vi "Build DashBoard Data.vi"(11 "Dashboard Enables":T2={"Analog Module 1"=[TRUE, TRUE, TRUE, TRUE, TRUE, TRUE, TRUE, TRUE], "Analog Module 2"=[FALSE, FALSE, FALSE, FALSE, FALSE, FALSE, FALSE, FALSE], "Digital Module 1"=TRUE, "Digital Module 2"=FALSE, "Solenoid Module"=TRUE}) -> ()   [LabVIEW 2011]
doc: "This VI builds data and sends it back to the dashboard PC program. By default it sends back the raw values for the first analog, digital, and solenoid module. Modify it to send back the data you want to view. Consider adding higher level data to the Dashboard Datatype.ctl and to this VI. Then update the Dashboard to display the data however you like.\n\nThis software is licensed. Open the labview\\readme\\WPI Robotics Library Open Source License.txt file for more information."
uses:
  DashboardEnable.ctl
  Dashboard Datatype.ctl
  <vilib>/Rock Robotics/WPI/DriverStation/WPI_DriverStationDigitalData.ctl
  System Set Points and States.vi
panel:
  out "Dashboard Data":T1
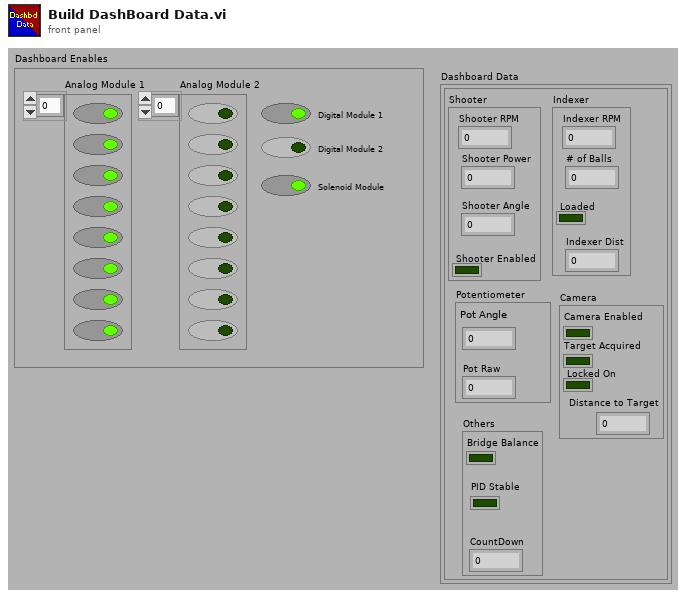
[diagram p1: front panel]
types:
  T1 = typedef "Dashboard Datatype.ctl" = cluster{"Robot Outputs":cluster{"Shooter":cluster{"Shooter RPM":dbl, "Shooter Angle":dbl, "Shooter Power":dbl, "Shooter Enabled":bool}, "Indexer":cluster{"Indexer RPM":dbl, "Loaded":bool, "# of Balls":dbl, "Indexer Dist":dbl}, "Camera":cluster{"Locked On":bool, "Target Acquired":bool, "Camera Enabled":bool, "Distance to Target":dbl}, "Potentiometer":cluster{"Pot Raw":dbl, "Pot Angle":dbl}, "Others":cluster{"CountDown":dbl, "Bridge Balance":bool, "PID Stable":bool}}}
  T2 = typedef "DashboardEnable.ctl" = cluster{"Analog Module 1":bool[], "Analog Module 2":bool[], "Digital Module 1":bool, "Digital Module 2":bool, "Solenoid Module":bool}
  T3 = typedef "WPI_DriverStationDigitalData.ctl" = cluster{"Relay Fwd":u8, "Relay Rev":u8, "GPIO":u16, "GPIO_OE":u16, "PWM":cluster{"PWM[0]":u8, "PWM[1]":u8, "PWM[2]":u8, "PWM[3]":u8, "PWM[4]":u8, "PWM[5]":u8, "PWM[6]":u8, "PWM[7]":u8, "PWM[8]":u8, "PWM[9]":u8}}
  T4 = cluster{"Shooter":cluster{"Shooter RPM":dbl, "Shooter Angle":dbl, "Shooter Power":dbl, "Shooter Enabled":bool}, "Indexer":cluster{"Indexer RPM":dbl, "Loaded":bool, "# of Balls":dbl, "Indexer Dist":dbl}, "Camera":cluster{"Locked On":bool, "Target Acquired":bool, "Camera Enabled":bool, "Distance to Target":dbl}, "Potentiometer":cluster{"Pot Raw":dbl, "Pot Angle":dbl}, "Others":cluster{"CountDown":dbl, "Bridge Balance":bool, "PID Stable":bool}}
  T5 = cluster{"Shooter RPM":dbl, "Shooter Angle":dbl, "Shooter Power":dbl, "Shooter Enabled":bool}
  T6 = cluster{"Indexer RPM":dbl, "Loaded":bool, "# of Balls":dbl, "Indexer Dist":dbl}
  T7 = cluster{"Locked On":bool, "Target Acquired":bool, "Camera Enabled":bool, "Distance to Target":dbl}
  T8 = cluster{"CountDown":dbl, "Bridge Balance":bool, "PID Stable":bool}
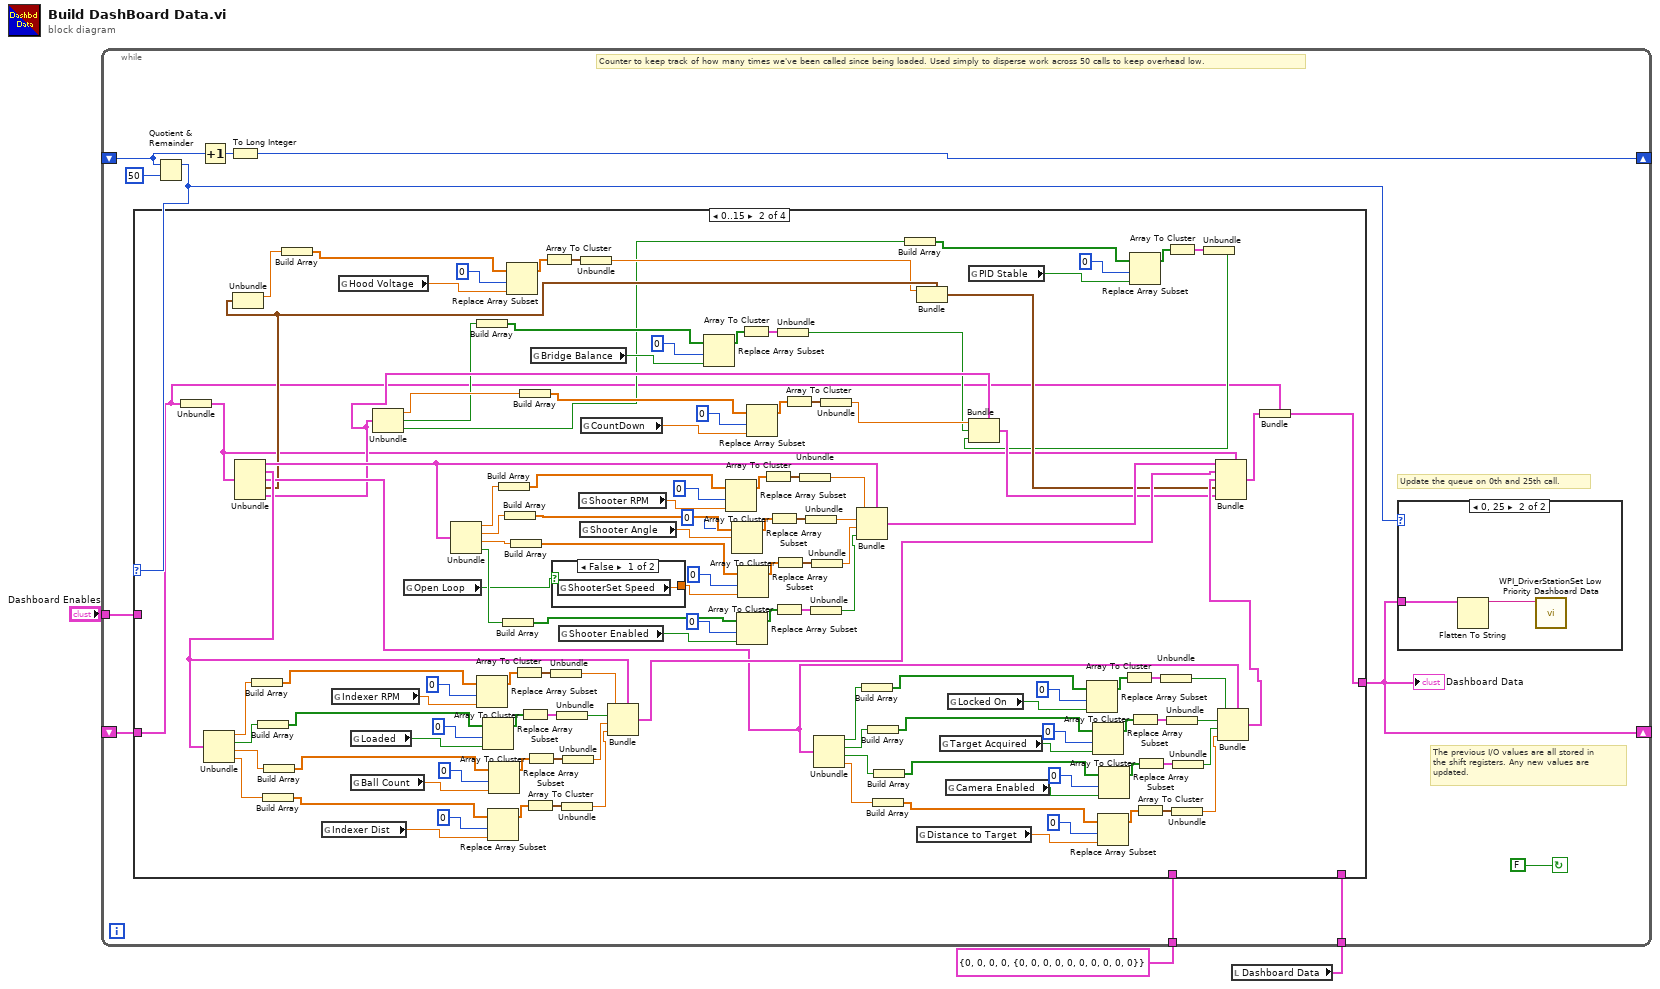
[diagram p0: block diagram]
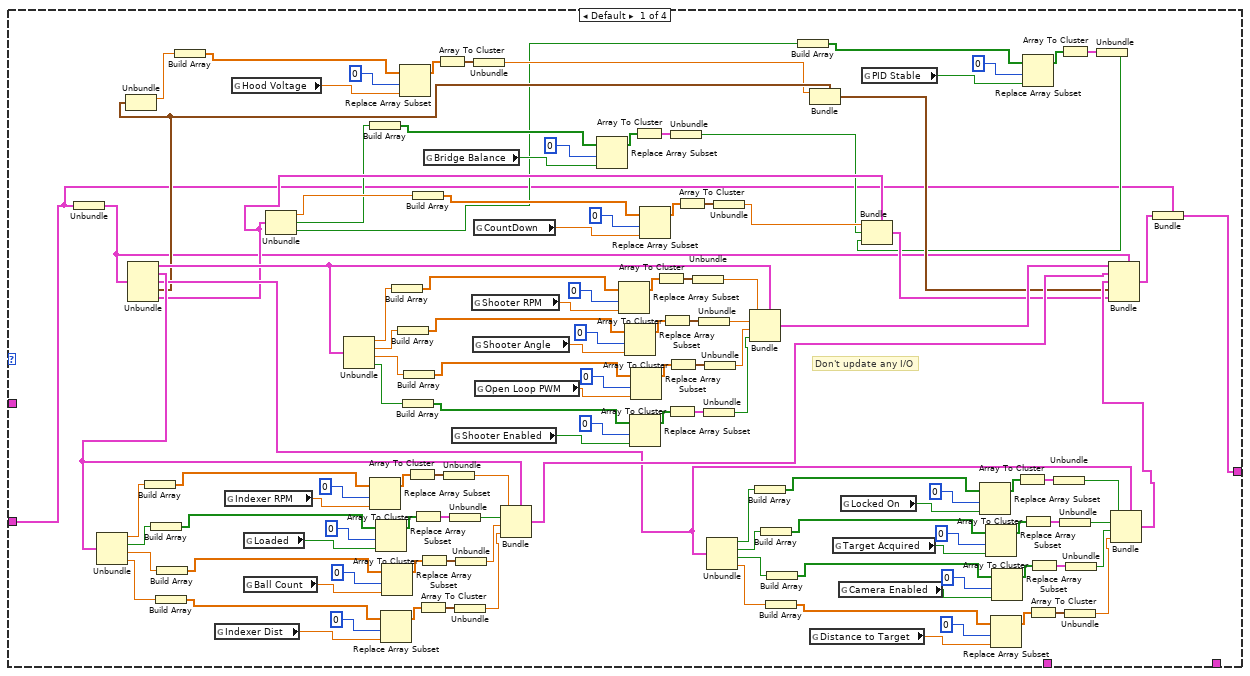
[diagram p3: hidden frame]
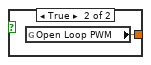
[diagram p4: hidden frame]
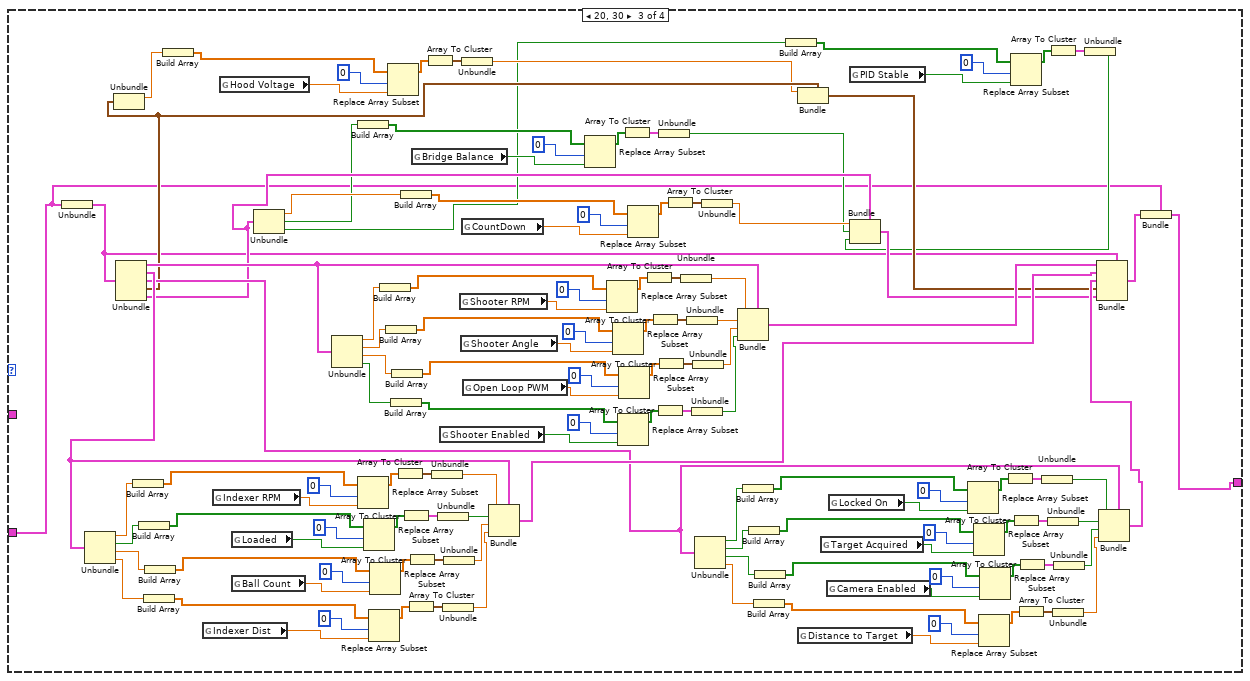
[diagram p5: hidden frame]
diagram:
  n1 = local read "Dashboard Data"() -> (w2:T1)
  n2 = while {
    shift-right: [w7] -> _
    shift-left: _ -> [w9]
    shift-right: [w4] -> _
    shift-left: _ -> [w12]
    tunnel: T3 {"Relay Fwd"=0, "Relay Rev"=0, "GPIO"=0, "GPIO_OE"=0, "PWM"={"PWM[0]"=0, "PWM[1]"=0, "PWM[2]"=0, "PWM[3]"=0, "PWM[4]"=0, "PWM[5]"=0, "PWM[6]"=0, "PWM[7]"=0, "PWM[8]"=0, "PWM[9]"=0}} ("DigitalModule[1]") -> [w11]
    tunnel: w2 -> [w6]
    tunnel: "Dashboard Enables" -> [w5]
    stop <- FALSE continue-if-true
    # "Counter to keep track of how many times we've been called since being loaded. Used simply to disperse work across 50 calls to keep overhead low."
    # "Update the queue on 0th and 25th call."
    # "The previous I/O values are all stored in\nthe shift registers. Any new values are\nupdated."
    n3 = Quotient & Remainder(x=w9, y=50) -> (x-y*floor(x/y)=w8:i32)  [unwired: 1 out]
    n4 = case shown="0..15" w8 {
      tunnel: [w17 w147 w272 w398] -> w4
      tunnel: w12 -> [w18 w146 w273 _]
      tunnel: w11 -> [_ _ _ _]
      tunnel: w6 -> [_ _ _ w398]
      tunnel: w5 -> [_ _ _ _]
      frame Default {
        # "Don't update any I/O"
        n5 = Unbundle(w18) -> ("Robot Outputs"=w20:T4)
        n6 = Unbundle(w20) -> ("Shooter"=w141:T5, "Indexer"=w84:T6, "Camera"=w54:T7, "Potentiometer"=w31:cluster{"Pot Raw":dbl, "Pot Angle":dbl}, "Others"=w46:T8)
        n7 = Unbundle(w84) -> ("Indexer RPM"=w106:dbl, "Loaded"=w100:bool, "# of Balls"=w92:dbl, "Indexer Dist"=w86:dbl)
        n8 = Unbundle(w31) -> ("Pot Raw"=w32:dbl)  [unwired: 1 out]
        n9 = Build Array(w106) -> (w112:dbl[])
        n10 = Build Array(w100) -> (w105:bool[])
        n11 = Build Array(w86) -> (w91:dbl[])
        n12 = Build Array(w92) -> (w98:dbl[])
        n13 = Build Array(w32) -> (w37:dbl[])
        n14 = global read "System Set Points and States.vi" "Indexer Dist"() -> (w89:dbl)
        n15 = global read "System Set Points and States.vi" "Indexer RPM"() -> (w109:dbl)
        n16 = global read "System Set Points and States.vi" "Hood Voltage"() -> (w35:dbl)
        n17 = global read "System Set Points and States.vi" "Loaded"() -> (w103:bool)
        n18 = global read "System Set Points and States.vi" "Ball Count"() -> (w96:dbl)
        n19 = Unbundle(w46) -> ("CountDown"=w47:dbl, "Bridge Balance"=w39:bool, "PID Stable"=w21:bool)
        n20 = Unbundle(w141) -> ("Shooter RPM"=w134:dbl, "Shooter Angle"=w128:dbl, "Shooter Power"=w120:dbl, "Shooter Enabled"=w114:bool)
        n21 = Build Array(w39) -> (w44:bool[])
        n22 = Replace Array Subset(array=w112, new element=w109, index=0) -> (w107:dbl[])
        n23 = Replace Array Subset(array=w105, new element=w103, index=0) -> (w101:bool[])
        n24 = Replace Array Subset(array=w91, new element=w89, index=0) -> (w87:dbl[])
        n25 = Replace Array Subset(array=w98, new element=w96, index=0) -> (w94:dbl[])
        n26 = Build Array(w134) -> (w142:dbl[])
        n27 = Build Array(w128) -> (w133:dbl[])
        n28 = Replace Array Subset(array=w37, new element=w35, index=0) -> (w33:dbl[])
        n29 = Build Array(w114) -> (w119:bool[])
        n30 = Build Array(w120) -> (w126:dbl[])
        n31 = Array To Cluster(array=w107) -> (cluster=w111:cluster{"[0]":dbl})
        n32 = Build Array(w47) -> (w52:dbl[])
        n33 = Array To Cluster(array=w101) -> (cluster=w104:cluster{"[0]":bool})
        n34 = Array To Cluster(array=w87) -> (cluster=w90:cluster{"[0]":dbl})
        n35 = Array To Cluster(array=w94) -> (cluster=w97:cluster{"[0]":dbl})
        n36 = global read "System Set Points and States.vi" "Bridge Balance"() -> (w42:bool)
        n37 = Array To Cluster(array=w33) -> (cluster=w36:cluster{"[0]":dbl})
        n38 = Unbundle(w111) -> ("[0]"=w110:dbl)
        n39 = Unbundle(w104) -> ("[0]"=w99:bool)
        n40 = global read "System Set Points and States.vi" "Shooter Enabled"() -> (w117:bool)
        n41 = Unbundle(w90) -> ("[0]"=w85:dbl)
        n42 = Unbundle(w97) -> ("[0]"=w93:dbl)
        n43 = global read "System Set Points and States.vi" "Shooter RPM"() -> (w137:dbl)
        n44 = global read "System Set Points and States.vi" "Shooter Angle"() -> (w131:dbl)
        n45 = Unbundle(w36) -> ("[0]"=w30:dbl)
        n46 = global read "System Set Points and States.vi" "CountDown"() -> (w50:dbl)
        n47 = global read "System Set Points and States.vi" "Open Loop PWM"() -> (w124:dbl)
        n48 = Bundle(cluster=w84, "Indexer RPM"=w110, "Loaded"=w99, "# of Balls"=w93, "Indexer Dist"=w85) -> (w83:T6)
        n49 = Replace Array Subset(array=w44, new element=w42, index=0) -> (w40:bool[])
        n50 = Replace Array Subset(array=w142, new element=w137, index=0) -> (w135:dbl[])
        n51 = Replace Array Subset(array=w133, new element=w131, index=0) -> (w129:dbl[])
        n52 = Replace Array Subset(array=w119, new element=w117, index=0) -> (w115:bool[])
        n53 = Replace Array Subset(array=w126, new element=w124, index=0) -> (w122:dbl[])
        n54 = Array To Cluster(array=w40) -> (cluster=w43:cluster{"[0]":bool})
        n55 = Replace Array Subset(array=w52, new element=w50, index=0) -> (w48:dbl[])
        n56 = Array To Cluster(array=w135) -> (cluster=w140:cluster{"[0]":dbl})
        n57 = Array To Cluster(array=w129) -> (cluster=w132:cluster{"[0]":dbl})
        n58 = Array To Cluster(array=w115) -> (cluster=w118:cluster{"[0]":bool})
        n59 = Array To Cluster(array=w122) -> (cluster=w125:cluster{"[0]":dbl})
        n60 = Unbundle(w43) -> ("[0]"=w38:bool)
        n61 = Array To Cluster(array=w48) -> (cluster=w51:cluster{"[0]":dbl})
        n62 = Unbundle(w140) -> ("[0]"=w139:dbl)
        n63 = Unbundle(w132) -> ("[0]"=w127:dbl)
        n64 = Unbundle(w118) -> ("[0]"=w113:bool)
        n65 = Unbundle(w125) -> ("[0]"=w121:dbl)
        n66 = Unbundle(w54) -> ("Locked On"=w76:bool, "Target Acquired"=w70:bool, "Camera Enabled"=w62:bool, "Distance to Target"=w56:dbl)
        n67 = Unbundle(w51) -> ("[0]"=w45:dbl)
        n68 = Bundle(cluster=w141, "Shooter RPM"=w139, "Shooter Angle"=w127, "Shooter Power"=w121, "Shooter Enabled"=w113) -> (w138:T5)
        n69 = Build Array(w76) -> (w82:bool[])
        n70 = Build Array(w70) -> (w75:bool[])
        n71 = Build Array(w56) -> (w61:dbl[])
        n72 = Build Array(w62) -> (w68:bool[])
        n73 = Build Array(w21) -> (w27:bool[])
        n74 = Bundle(cluster=w31, "Pot Raw"=w30) -> (w29:cluster{"Pot Raw":dbl, "Pot Angle":dbl})  [unwired: 1 in]
        n75 = global read "System Set Points and States.vi" "Distance to Target"() -> (w59:dbl)
        n76 = global read "System Set Points and States.vi" "Target Acquired"() -> (w73:bool)
        n77 = global read "System Set Points and States.vi" "Camera Enabled"() -> (w66:bool)
        n78 = global read "System Set Points and States.vi" "Locked On"() -> (w79:bool)
        n79 = global read "System Set Points and States.vi" "PID Stable"() -> (w25:bool)
        n80 = Replace Array Subset(array=w82, new element=w79, index=0) -> (w77:bool[])
        n81 = Replace Array Subset(array=w75, new element=w73, index=0) -> (w71:bool[])
        n82 = Replace Array Subset(array=w61, new element=w59, index=0) -> (w57:dbl[])
        n83 = Replace Array Subset(array=w68, new element=w66, index=0) -> (w64:bool[])
        n84 = Array To Cluster(array=w77) -> (cluster=w81:cluster{"[0]":bool})
        n85 = Replace Array Subset(array=w27, new element=w25, index=0) -> (w23:bool[])
        n86 = Array To Cluster(array=w71) -> (cluster=w74:cluster{"[0]":bool})
        n87 = Array To Cluster(array=w57) -> (cluster=w60:cluster{"[0]":dbl})
        n88 = Array To Cluster(array=w64) -> (cluster=w67:cluster{"[0]":bool})
        n89 = Unbundle(w81) -> ("[0]"=w80:bool)
        n90 = Array To Cluster(array=w23) -> (cluster=w26:cluster{"[0]":bool})
        n91 = Unbundle(w74) -> ("[0]"=w69:bool)
        n92 = Unbundle(w60) -> ("[0]"=w55:dbl)
        n93 = Unbundle(w67) -> ("[0]"=w63:bool)
        n94 = Unbundle(w26) -> ("[0]"=w22:bool)
        n95 = Bundle(cluster=w46, "CountDown"=w45, "Bridge Balance"=w38, "PID Stable"=w22) -> (w28:T8)
        n96 = Bundle(cluster=w54, "Locked On"=w80, "Target Acquired"=w69, "Camera Enabled"=w63, "Distance to Target"=w55) -> (w53:T7)
        n97 = Bundle(cluster=w20, "Shooter"=w138, "Indexer"=w83, "Camera"=w53, "Potentiometer"=w29, "Others"=w28) -> (w19:T4)
        n98 = Bundle(cluster=w18, "Robot Outputs"=w19) -> (w17:T1)
      }
      frame 0..15 {
        n99 = Unbundle(w146) -> ("Robot Outputs"=w145:T4)
        n100 = Unbundle(w145) -> ("Shooter"=w268:T5, "Indexer"=w211:T6, "Camera"=w181:T7, "Potentiometer"=w158:cluster{"Pot Raw":dbl, "Pot Angle":dbl}, "Others"=w173:T8)
        n101 = Unbundle(w211) -> ("Indexer RPM"=w233:dbl, "Loaded"=w227:bool, "# of Balls"=w219:dbl, "Indexer Dist"=w213:dbl)
        n102 = Unbundle(w158) -> ("Pot Raw"=w159:dbl)  [unwired: 1 out]
        n103 = Build Array(w233) -> (w239:dbl[])
        n104 = Build Array(w227) -> (w232:bool[])
        n105 = Build Array(w213) -> (w218:dbl[])
        n106 = Build Array(w219) -> (w225:dbl[])
        n107 = Build Array(w159) -> (w164:dbl[])
        n108 = global read "System Set Points and States.vi" "Indexer Dist"() -> (w216:dbl)
        n109 = global read "System Set Points and States.vi" "Indexer RPM"() -> (w236:dbl)
        n110 = global read "System Set Points and States.vi" "Hood Voltage"() -> (w162:dbl)
        n111 = global read "System Set Points and States.vi" "Loaded"() -> (w230:bool)
        n112 = global read "System Set Points and States.vi" "Ball Count"() -> (w223:dbl)
        n113 = Unbundle(w173) -> ("CountDown"=w174:dbl, "Bridge Balance"=w166:bool, "PID Stable"=w148:bool)
        n114 = global read "System Set Points and States.vi" "Open Loop"() -> (w143:bool)
        n115 = Unbundle(w268) -> ("Shooter RPM"=w261:dbl, "Shooter Angle"=w255:dbl, "Shooter Power"=w247:dbl, "Shooter Enabled"=w241:bool)
        n116 = Build Array(w166) -> (w171:bool[])
        n117 = Replace Array Subset(array=w239, new element=w236, index=0) -> (w234:dbl[])
        n118 = Replace Array Subset(array=w232, new element=w230, index=0) -> (w228:bool[])
        n119 = Replace Array Subset(array=w218, new element=w216, index=0) -> (w214:dbl[])
        n120 = Replace Array Subset(array=w225, new element=w223, index=0) -> (w221:dbl[])
        n121 = Build Array(w261) -> (w269:dbl[])
        n122 = Build Array(w241) -> (w246:bool[])
        n123 = Build Array(w255) -> (w260:dbl[])
        n124 = Replace Array Subset(array=w164, new element=w162, index=0) -> (w160:dbl[])
        n125 = Build Array(w247) -> (w253:dbl[])
        n126 = Array To Cluster(array=w234) -> (cluster=w238:cluster{"[0]":dbl})
        n127 = Build Array(w174) -> (w179:dbl[])
        n128 = Array To Cluster(array=w228) -> (cluster=w231:cluster{"[0]":bool})
        n129 = Array To Cluster(array=w214) -> (cluster=w217:cluster{"[0]":dbl})
        n130 = Array To Cluster(array=w221) -> (cluster=w224:cluster{"[0]":dbl})
        n131 = global read "System Set Points and States.vi" "Bridge Balance"() -> (w169:bool)
        n132 = Array To Cluster(array=w160) -> (cluster=w163:cluster{"[0]":dbl})
        n133 = Unbundle(w238) -> ("[0]"=w237:dbl)
        n134 = case shown="False" w143 {
          tunnel: [w270 w271] -> w251
          frame False {
            n135 = global read "System Set Points and States.vi" "ShooterSet Speed"() -> (w270:dbl)
          }
          frame True {
            n136 = global read "System Set Points and States.vi" "Open Loop PWM"() -> (w271:dbl)
          }
        }
        n137 = Unbundle(w231) -> ("[0]"=w226:bool)
        n138 = global read "System Set Points and States.vi" "Shooter Enabled"() -> (w244:bool)
        n139 = Unbundle(w217) -> ("[0]"=w212:dbl)
        n140 = Unbundle(w224) -> ("[0]"=w220:dbl)
        n141 = global read "System Set Points and States.vi" "Shooter RPM"() -> (w264:dbl)
        n142 = global read "System Set Points and States.vi" "Shooter Angle"() -> (w258:dbl)
        n143 = Unbundle(w163) -> ("[0]"=w157:dbl)
        n144 = global read "System Set Points and States.vi" "CountDown"() -> (w177:dbl)
        n145 = Bundle(cluster=w211, "Indexer RPM"=w237, "Loaded"=w226, "# of Balls"=w220, "Indexer Dist"=w212) -> (w210:T6)
        n146 = Replace Array Subset(array=w171, new element=w169, index=0) -> (w167:bool[])
        n147 = Replace Array Subset(array=w269, new element=w264, index=0) -> (w262:dbl[])
        n148 = Replace Array Subset(array=w260, new element=w258, index=0) -> (w256:dbl[])
        n149 = Replace Array Subset(array=w246, new element=w244, index=0) -> (w242:bool[])
        n150 = Replace Array Subset(array=w253, new element=w251, index=0) -> (w249:dbl[])
        n151 = Array To Cluster(array=w167) -> (cluster=w170:cluster{"[0]":bool})
        n152 = Replace Array Subset(array=w179, new element=w177, index=0) -> (w175:dbl[])
        n153 = Array To Cluster(array=w262) -> (cluster=w267:cluster{"[0]":dbl})
        n154 = Array To Cluster(array=w256) -> (cluster=w259:cluster{"[0]":dbl})
        n155 = Array To Cluster(array=w242) -> (cluster=w245:cluster{"[0]":bool})
        n156 = Array To Cluster(array=w249) -> (cluster=w252:cluster{"[0]":dbl})
        n157 = Unbundle(w170) -> ("[0]"=w165:bool)
        n158 = Array To Cluster(array=w175) -> (cluster=w178:cluster{"[0]":dbl})
        n159 = Unbundle(w267) -> ("[0]"=w266:dbl)
        n160 = Unbundle(w259) -> ("[0]"=w254:dbl)
        n161 = Unbundle(w245) -> ("[0]"=w240:bool)
        n162 = Unbundle(w252) -> ("[0]"=w248:dbl)
        n163 = Unbundle(w181) -> ("Locked On"=w203:bool, "Target Acquired"=w197:bool, "Camera Enabled"=w189:bool, "Distance to Target"=w183:dbl)
        n164 = Unbundle(w178) -> ("[0]"=w172:dbl)
        n165 = Bundle(cluster=w268, "Shooter RPM"=w266, "Shooter Angle"=w254, "Shooter Power"=w248, "Shooter Enabled"=w240) -> (w265:T5)
        n166 = Build Array(w203) -> (w209:bool[])
        n167 = Build Array(w197) -> (w202:bool[])
        n168 = Build Array(w183) -> (w188:dbl[])
        n169 = Build Array(w189) -> (w195:bool[])
        n170 = Build Array(w148) -> (w154:bool[])
        n171 = Bundle(cluster=w158, "Pot Raw"=w157) -> (w156:cluster{"Pot Raw":dbl, "Pot Angle":dbl})  [unwired: 1 in]
        n172 = global read "System Set Points and States.vi" "Distance to Target"() -> (w186:dbl)
        n173 = global read "System Set Points and States.vi" "Target Acquired"() -> (w200:bool)
        n174 = global read "System Set Points and States.vi" "Camera Enabled"() -> (w193:bool)
        n175 = global read "System Set Points and States.vi" "Locked On"() -> (w206:bool)
        n176 = global read "System Set Points and States.vi" "PID Stable"() -> (w152:bool)
        n177 = Replace Array Subset(array=w209, new element=w206, index=0) -> (w204:bool[])
        n178 = Replace Array Subset(array=w202, new element=w200, index=0) -> (w198:bool[])
        n179 = Replace Array Subset(array=w188, new element=w186, index=0) -> (w184:dbl[])
        n180 = Replace Array Subset(array=w195, new element=w193, index=0) -> (w191:bool[])
        n181 = Array To Cluster(array=w204) -> (cluster=w208:cluster{"[0]":bool})
        n182 = Replace Array Subset(array=w154, new element=w152, index=0) -> (w150:bool[])
        n183 = Array To Cluster(array=w198) -> (cluster=w201:cluster{"[0]":bool})
        n184 = Array To Cluster(array=w184) -> (cluster=w187:cluster{"[0]":dbl})
        n185 = Array To Cluster(array=w191) -> (cluster=w194:cluster{"[0]":bool})
        n186 = Unbundle(w208) -> ("[0]"=w207:bool)
        n187 = Array To Cluster(array=w150) -> (cluster=w153:cluster{"[0]":bool})
        n188 = Unbundle(w201) -> ("[0]"=w196:bool)
        n189 = Unbundle(w187) -> ("[0]"=w182:dbl)
        n190 = Unbundle(w194) -> ("[0]"=w190:bool)
        n191 = Unbundle(w153) -> ("[0]"=w149:bool)
        n192 = Bundle(cluster=w173, "CountDown"=w172, "Bridge Balance"=w165, "PID Stable"=w149) -> (w155:T8)
        n193 = Bundle(cluster=w181, "Locked On"=w207, "Target Acquired"=w196, "Camera Enabled"=w190, "Distance to Target"=w182) -> (w180:T7)
        n194 = Bundle(cluster=w145, "Shooter"=w265, "Indexer"=w210, "Camera"=w180, "Potentiometer"=w156, "Others"=w155) -> (w144:T4)
        n195 = Bundle(cluster=w146, "Robot Outputs"=w144) -> (w147:T1)
      }
      frame 20, 30 {
        n196 = Unbundle(w273) -> ("Robot Outputs"=w275:T4)
        n197 = Unbundle(w275) -> ("Shooter"=w396:T5, "Indexer"=w339:T6, "Camera"=w309:T7, "Potentiometer"=w286:cluster{"Pot Raw":dbl, "Pot Angle":dbl}, "Others"=w301:T8)
        n198 = Unbundle(w339) -> ("Indexer RPM"=w361:dbl, "Loaded"=w355:bool, "# of Balls"=w347:dbl, "Indexer Dist"=w341:dbl)
        n199 = Unbundle(w286) -> ("Pot Raw"=w287:dbl)  [unwired: 1 out]
        n200 = Build Array(w361) -> (w367:dbl[])
        n201 = Build Array(w355) -> (w360:bool[])
        n202 = Build Array(w341) -> (w346:dbl[])
        n203 = Build Array(w347) -> (w353:dbl[])
        n204 = Build Array(w287) -> (w292:dbl[])
        n205 = global read "System Set Points and States.vi" "Indexer Dist"() -> (w344:dbl)
        n206 = global read "System Set Points and States.vi" "Indexer RPM"() -> (w364:dbl)
        n207 = global read "System Set Points and States.vi" "Hood Voltage"() -> (w290:dbl)
        n208 = global read "System Set Points and States.vi" "Loaded"() -> (w358:bool)
        n209 = global read "System Set Points and States.vi" "Ball Count"() -> (w351:dbl)
        n210 = Unbundle(w301) -> ("CountDown"=w302:dbl, "Bridge Balance"=w294:bool, "PID Stable"=w276:bool)
        n211 = Unbundle(w396) -> ("Shooter RPM"=w389:dbl, "Shooter Angle"=w383:dbl, "Shooter Power"=w375:dbl, "Shooter Enabled"=w369:bool)
        n212 = Build Array(w294) -> (w299:bool[])
        n213 = Replace Array Subset(array=w367, new element=w364, index=0) -> (w362:dbl[])
        n214 = Replace Array Subset(array=w360, new element=w358, index=0) -> (w356:bool[])
        n215 = Replace Array Subset(array=w346, new element=w344, index=0) -> (w342:dbl[])
        n216 = Replace Array Subset(array=w353, new element=w351, index=0) -> (w349:dbl[])
        n217 = Build Array(w389) -> (w397:dbl[])
        n218 = Build Array(w383) -> (w388:dbl[])
        n219 = Replace Array Subset(array=w292, new element=w290, index=0) -> (w288:dbl[])
        n220 = Build Array(w369) -> (w374:bool[])
        n221 = Build Array(w375) -> (w381:dbl[])
        n222 = Array To Cluster(array=w362) -> (cluster=w366:cluster{"[0]":dbl})
        n223 = Build Array(w302) -> (w307:dbl[])
        n224 = Array To Cluster(array=w356) -> (cluster=w359:cluster{"[0]":bool})
        n225 = Array To Cluster(array=w342) -> (cluster=w345:cluster{"[0]":dbl})
        n226 = Array To Cluster(array=w349) -> (cluster=w352:cluster{"[0]":dbl})
        n227 = global read "System Set Points and States.vi" "Bridge Balance"() -> (w297:bool)
        n228 = Array To Cluster(array=w288) -> (cluster=w291:cluster{"[0]":dbl})
        n229 = Unbundle(w366) -> ("[0]"=w365:dbl)
        n230 = Unbundle(w359) -> ("[0]"=w354:bool)
        n231 = global read "System Set Points and States.vi" "Shooter Enabled"() -> (w372:bool)
        n232 = Unbundle(w345) -> ("[0]"=w340:dbl)
        n233 = Unbundle(w352) -> ("[0]"=w348:dbl)
        n234 = global read "System Set Points and States.vi" "Shooter RPM"() -> (w392:dbl)
        n235 = global read "System Set Points and States.vi" "Shooter Angle"() -> (w386:dbl)
        n236 = Unbundle(w291) -> ("[0]"=w285:dbl)
        n237 = global read "System Set Points and States.vi" "CountDown"() -> (w305:dbl)
        n238 = global read "System Set Points and States.vi" "Open Loop PWM"() -> (w379:dbl)
        n239 = Bundle(cluster=w339, "Indexer RPM"=w365, "Loaded"=w354, "# of Balls"=w348, "Indexer Dist"=w340) -> (w338:T6)
        n240 = Replace Array Subset(array=w299, new element=w297, index=0) -> (w295:bool[])
        n241 = Replace Array Subset(array=w397, new element=w392, index=0) -> (w390:dbl[])
        n242 = Replace Array Subset(array=w388, new element=w386, index=0) -> (w384:dbl[])
        n243 = Replace Array Subset(array=w374, new element=w372, index=0) -> (w370:bool[])
        n244 = Replace Array Subset(array=w381, new element=w379, index=0) -> (w377:dbl[])
        n245 = Array To Cluster(array=w295) -> (cluster=w298:cluster{"[0]":bool})
        n246 = Replace Array Subset(array=w307, new element=w305, index=0) -> (w303:dbl[])
        n247 = Array To Cluster(array=w390) -> (cluster=w395:cluster{"[0]":dbl})
        n248 = Array To Cluster(array=w384) -> (cluster=w387:cluster{"[0]":dbl})
        n249 = Array To Cluster(array=w370) -> (cluster=w373:cluster{"[0]":bool})
        n250 = Array To Cluster(array=w377) -> (cluster=w380:cluster{"[0]":dbl})
        n251 = Unbundle(w298) -> ("[0]"=w293:bool)
        n252 = Array To Cluster(array=w303) -> (cluster=w306:cluster{"[0]":dbl})
        n253 = Unbundle(w395) -> ("[0]"=w394:dbl)
        n254 = Unbundle(w387) -> ("[0]"=w382:dbl)
        n255 = Unbundle(w373) -> ("[0]"=w368:bool)
        n256 = Unbundle(w380) -> ("[0]"=w376:dbl)
        n257 = Unbundle(w309) -> ("Locked On"=w331:bool, "Target Acquired"=w325:bool, "Camera Enabled"=w317:bool, "Distance to Target"=w311:dbl)
        n258 = Unbundle(w306) -> ("[0]"=w300:dbl)
        n259 = Bundle(cluster=w396, "Shooter RPM"=w394, "Shooter Angle"=w382, "Shooter Power"=w376, "Shooter Enabled"=w368) -> (w393:T5)
        n260 = Build Array(w331) -> (w337:bool[])
        n261 = Build Array(w325) -> (w330:bool[])
        n262 = Build Array(w311) -> (w316:dbl[])
        n263 = Build Array(w317) -> (w323:bool[])
        n264 = Build Array(w276) -> (w282:bool[])
        n265 = Bundle(cluster=w286, "Pot Raw"=w285) -> (w284:cluster{"Pot Raw":dbl, "Pot Angle":dbl})  [unwired: 1 in]
        n266 = global read "System Set Points and States.vi" "Distance to Target"() -> (w314:dbl)
        n267 = global read "System Set Points and States.vi" "Target Acquired"() -> (w328:bool)
        n268 = global read "System Set Points and States.vi" "Camera Enabled"() -> (w321:bool)
        n269 = global read "System Set Points and States.vi" "Locked On"() -> (w334:bool)
        n270 = global read "System Set Points and States.vi" "PID Stable"() -> (w280:bool)
        n271 = Replace Array Subset(array=w337, new element=w334, index=0) -> (w332:bool[])
        n272 = Replace Array Subset(array=w330, new element=w328, index=0) -> (w326:bool[])
        n273 = Replace Array Subset(array=w316, new element=w314, index=0) -> (w312:dbl[])
        n274 = Replace Array Subset(array=w323, new element=w321, index=0) -> (w319:bool[])
        n275 = Array To Cluster(array=w332) -> (cluster=w336:cluster{"[0]":bool})
        n276 = Replace Array Subset(array=w282, new element=w280, index=0) -> (w278:bool[])
        n277 = Array To Cluster(array=w326) -> (cluster=w329:cluster{"[0]":bool})
        n278 = Array To Cluster(array=w312) -> (cluster=w315:cluster{"[0]":dbl})
        n279 = Array To Cluster(array=w319) -> (cluster=w322:cluster{"[0]":bool})
        n280 = Unbundle(w336) -> ("[0]"=w335:bool)
        n281 = Array To Cluster(array=w278) -> (cluster=w281:cluster{"[0]":bool})
        n282 = Unbundle(w329) -> ("[0]"=w324:bool)
        n283 = Unbundle(w315) -> ("[0]"=w310:dbl)
        n284 = Unbundle(w322) -> ("[0]"=w318:bool)
        n285 = Unbundle(w281) -> ("[0]"=w277:bool)
        n286 = Bundle(cluster=w301, "CountDown"=w300, "Bridge Balance"=w293, "PID Stable"=w277) -> (w283:T8)
        n287 = Bundle(cluster=w309, "Locked On"=w335, "Target Acquired"=w324, "Camera Enabled"=w318, "Distance to Target"=w310) -> (w308:T7)
        n288 = Bundle(cluster=w275, "Shooter"=w393, "Indexer"=w338, "Camera"=w308, "Potentiometer"=w284, "Others"=w283) -> (w274:T4)
        n289 = Bundle(cluster=w273, "Robot Outputs"=w274) -> (w272:T1)
      }
      frame 40 {
      }
    }
    "Dashboard Data" <- w4
    n290 = Increment(x=w9) -> (x+1=w14:i32)
    n291 = To Long Integer(number=w14) -> (32bit integer=w7:i32)
    n292 = case shown="0, 25" w8 {
      tunnel: w4 -> [_ w16]
      frame Default {
      }
      frame 0, 25 {
        n293 = Flatten To String(anything=w16) -> (data string=w15:string)  [unwired: 1 in, 4 out]
        n294 = call <vilib>:"WPI_DriverStationSet Low Priority Dashboard Data.vi"("User Data"=w15) -> ()  [unwired: 1 in, 10 out]
      }
    }
  }
